vi "Get Configuration.vi"(11 "IConfigurable in":refnum<class "IConfigurable.lvclass">) -> (2 "IConfigure.lvclass":refnum<class "IConfigure.lvclass">, 3 "IConfigurable out":refnum<class "IConfigurable.lvclass">)   [LabVIEW 2024, in "IConfigurable.lvclass"]
uses:
  IConfigurable.lvclass
  IConfigure/IConfigure.lvclass
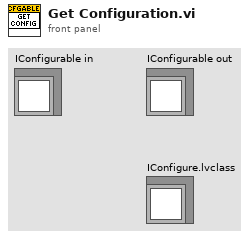
[diagram p1: front panel]
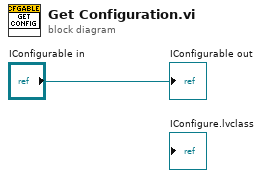
[diagram p0: block diagram]
diagram:
  "IConfigurable out" <- "IConfigurable in"
